vi "SENS_PATH_CONF_ELEM_VAL_CAT.vi"(0 "VISA IN":refnum<visa-resource-name>, 5 "error in":errorcluster, 7 "Switch":string) -> (13 "Data":string[](array[string]), 14 "VISA Out":refnum<visa-resource-name>, 19 "error out":errorcluster)   [LabVIEW 2018, in "PNA-X.lvlib"]
doc: "SENSe:PATH:CONFiguration:DELete <string>\n(Write-only) Deletes the specified configuration name from the PNA. The factory configurations cannot be deleted. This is the only method of distinguishing a factory configuration from a user-named configuration.\n \nParameters\n \n \n<string>\n Configuration name to be deleted.\n \nExamples\n SENS:PATH:CONF:DEL \"MyMixer\"\n \nReturn Type\n Not Applicable\n \nDefault\n Not Applicable"
uses:
  PNA-X.lvlib
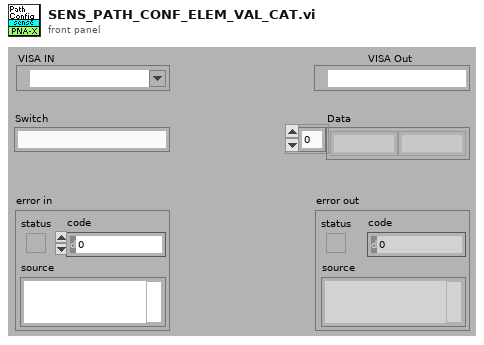
[diagram p1: front panel]
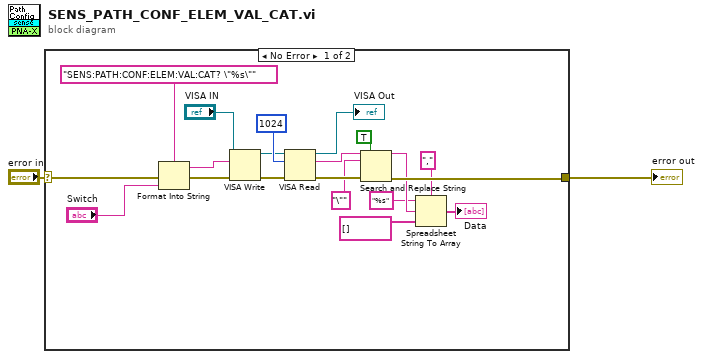
[diagram p0: block diagram]
diagram:
  n1 = case shown="No Error" "error in" {
    selector: "error in" -> [w6 w23]
    tunnel: [w16 w23] -> w1
    frame No Error {
      n2 = Format Into String(format string="SENS:PATH:CONF:ELEM:VAL:CAT? \"%s\"" ("Cmdline"), error in=w6, "Switch") -> (resulting string=w5:string, error out=w7:errorcluster)  [unwired: 1 in]
      n3 = VISA Write(VISA resource name="VISA IN", write buffer=w5, error in (no error)=w7) -> (VISA resource name out=w19:refnum<visa-resource-name>, error out=w21:errorcluster)  [unwired: 1 out]
      n4 = VISA Read(VISA resource name=w19, byte count=1024, error in (no error)=w21) -> (VISA resource name out=→"VISA Out":refnum<visa-resource-name>, read buffer=w15:string, error out=w17:errorcluster)  [unwired: 1 out]
      n5 = Search and Replace String(replace all?=TRUE ("replace all? (F)"), input string=w15, search string="\"", error in=w17) -> (result string=w12:string, error out=w16:errorcluster)  [unwired: 4 in, 2 out]
      n6 = Spreadsheet String To Array(delimiter (Tab)=",", format string="%s", spreadsheet string=w12, array type (2D Dbl)=string[] []) -> (array=→"Data":string[])
    }
    frame Error {
    }
  }
  "error out" <- w1
